vi "Route.vi"(8 "error in (no error)":errorcluster, 9 "Connect":bool, 10 "channel 1":string caption="Route", 11 "reference in":refnum<class "Switch_MotorP5.lvclass">) -> (0 "error out":errorcluster, 3 "reference in":refnum<class "Switch_MotorP5.lvclass">)   [LabVIEW 2022 SP3, in "Switch_MotorP5.lvlib" / "Switch_MotorP5.lvclass"]
uses:
  Switch_MotorP5.lvclass
  5b888fd5-fbae-499d-b477-1edb2fb80a14.vi
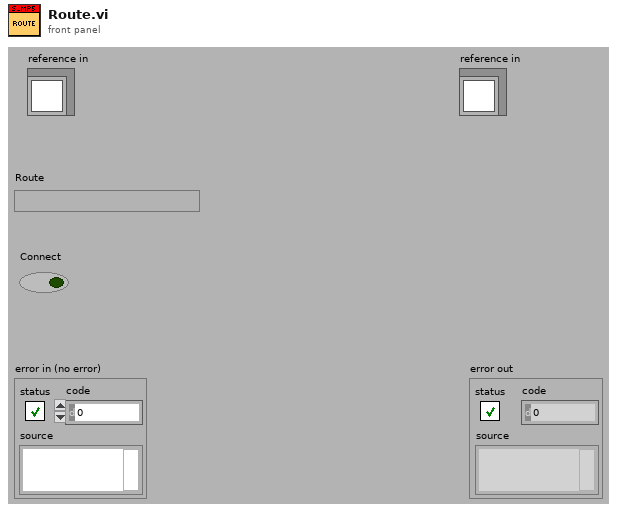
[diagram p1: front panel]
types:
  T1 = typedef "Switch_MotorP5.lvlib/Switch_MotorP5.lvclass/ObjectAttributes.ctl" = cluster{"Config":T2, "VISA":refnum<visa-resource-name>, "RPM":i32, "States":bool[], "UpdateEvent":refnum<user-event>, "Motor":enum32{"M1", "M2", "M3", "M4", "M5", "M6", "M7", "M8"}}
  T2 = typedef "Switch_MotorP5.lvlib/Switch_MotorP5.lvclass/Config.ctl" = cluster{"COM":refnum<visa-resource-name>, "SwitchMap":cluster{"Name":string, "Description":string, "Group":string, "IsGroup":bool, "Motor":enum32{"M1", "M2", "M3", "M4", "M5", "M6", "M7", "M8", "NA"}}[], "Sim":bool}
  T3 = cluster{"Name":string, "Description":string, "Group":string, "IsGroup":bool, "Motor":enum32{"M1", "M2", "M3", "M4", "M5", "M6", "M7", "M8", "NA"}}[]
  T4 = enum32{"M1", "M2", "M3", "M4", "M5", "M6", "M7", "M8", "NA"}
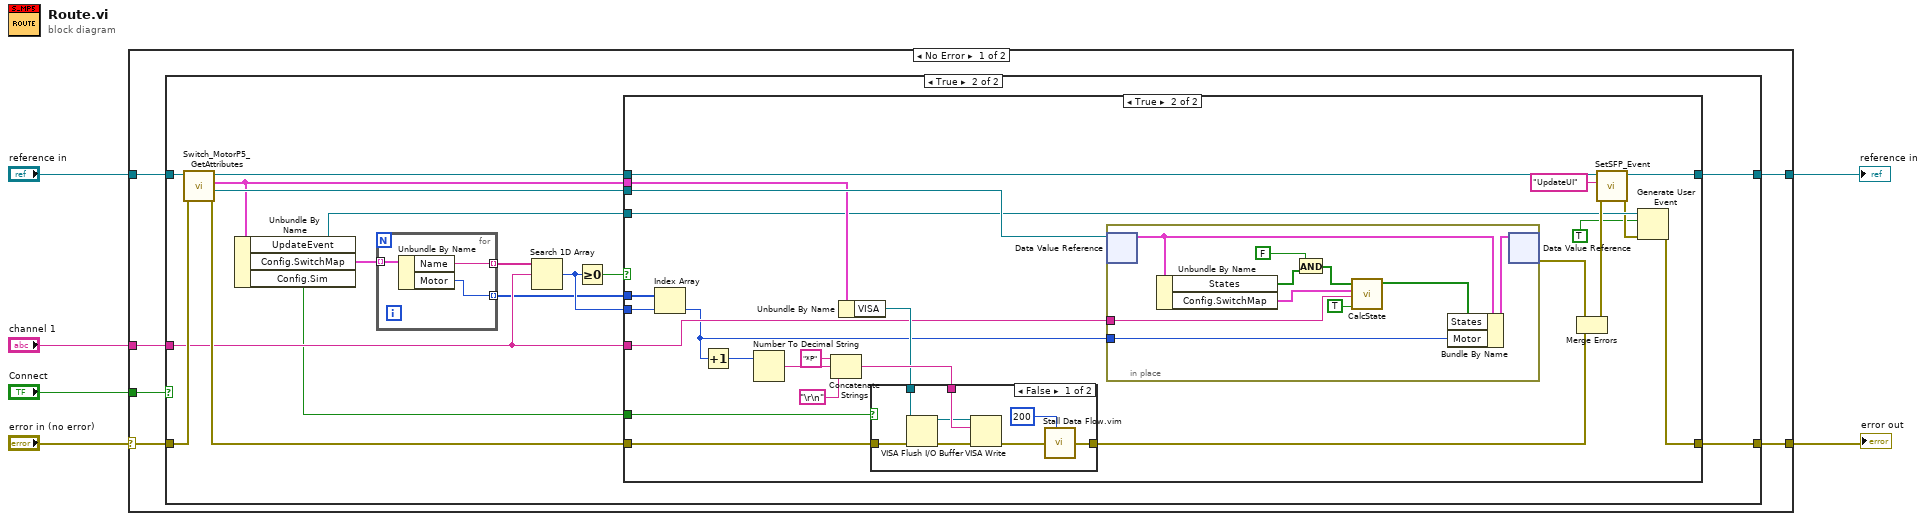
[diagram p0: block diagram]
diagram:
  n1 = case shown="No Error" "error in (no error)" {
    selector: "error in (no error)" -> [w11 w80]
    tunnel: [w8 w80] -> w5
    tunnel: [w9 w79] -> w3
    tunnel: "reference in" -> [w10 w79]
    tunnel: "channel 1" -> [w12 _]
    tunnel: "Connect" -> [w7 _]
    frame No Error {
      n2 = case shown="True" w7 {
        tunnel: w12 -> [_ w20]
        tunnel: w11 -> [w13 w30]
        tunnel: w10 -> [w14 w29]
        tunnel: [w14 w25] -> w9
        tunnel: [w13 w24] -> w8
        frame False {
        }
        frame True {
          n3 = call "Switch_MotorP5_GetAttributes.vi"("error in (no error)"=w30, "reference in"=w29) -> ("error out"=w28:errorcluster, "DataRef"=w27:refnum<data-value>, "Data"=w23:T1, "reference out"=w26:refnum<class "Switch_MotorP5.lvclass">)  [unwired: 6 in]
          n4 = Unbundle By Name(w23) -> ("UpdateEvent"=w15:refnum<user-event>, "Config.SwitchMap"=w22:T3, "Config.Sim"=w16:bool)
          n5 = for {
            tunnel: w22 -> [w78] mode=indexing
            tunnel: [w77] -> w21 mode=indexing
            tunnel: [w76] -> w17 mode=indexing
            n6 = Unbundle By Name(w78) -> ("Name"=w77:string, "Motor"=w76:T4)
          }
          n7 = Search 1D Array(1D array=w21, element=w20) -> (index of element=w18:i32)  [unwired: 1 in]
          n8 = Greater Or Equal To 0?(x=w18) -> (x >= 0?=w19:bool)
          n9 = case shown="True" w19 {
            tunnel: w28 -> [w32 w54]
            tunnel: w27 -> [_ w50]
            tunnel: w26 -> [w31 w49]
            tunnel: [w31 w48] -> w25
            tunnel: [w32 w37] -> w24
            tunnel: w23 -> [_ w43]
            tunnel: w20 -> [_ w35]
            tunnel: w18 -> [_ w42]
            tunnel: w17 -> [_ w41]
            tunnel: w16 -> [_ w40]
            tunnel: w15 -> [_ w39]
            frame False {
            }
            frame True {
              n10 = Index Array(array=w41, index=w42) -> (element=w34:T4)
              n11 = Increment(x=w34) -> (x+1=w33:T4)
              n12 = Number To Decimal String(number=w33) -> (decimal integer string=w56:string)  [unwired: 1 in]
              n13 = Concatenate Strings("*P" ("string"), w56, "\r\n") -> (w55:string)
              n14 = Unbundle By Name(w43) -> ("VISA"=w53:refnum<visa-resource-name>)
              n15 = case shown="False" w40 {
                tunnel: w55 -> [w64 _]
                tunnel: w54 -> [w63 w65]
                tunnel: w53 -> [w61 _]
                tunnel: [w58 w65] -> w44
                frame False {
                  n16 = VISA Flush I/O Buffer(VISA resource name=w61, error in (no error)=w63) -> (VISA resource name out=w60:refnum<visa-resource-name>, error out=w62:errorcluster)  [unwired: 1 in]
                  n17 = VISA Write(VISA resource name=w60, write buffer=w64, error in (no error)=w62) -> (error out=w59:errorcluster)  [unwired: 2 out]
                  n18 = call "Stall Data Flow.vim"("value in"=w59, "milliseconds to wait"=u32 200) -> ("value out"=w58:errorcluster)  [unwired: 1 out]
                }
                frame True {
                }
              }
              n19 = in-place {
                in-place-border: w34 -> [w73]
                in-place-border: w35 -> [w71]
                n20 = in-place-dvr #1(w50) -> (w74:T1)  [unwired: 1 out]
                n21 = Unbundle By Name(w74) -> ("States"=w67:bool[], "Config.SwitchMap"=w72:T3)
                n22 = And(x=FALSE ("State"), y=w67) -> (x .and. y?=w66:bool[])
                n23 = call "CalcState.vi"("State"=TRUE, "Item"=w71, "SwitchMap"=w72, "State_In"=w66) -> ("State_Out"=w69:bool[])  [unwired: 7 in]
                n24 = Bundle By Name(cluster=w74, "States"=w69, "Motor"=w73) -> (w75:T1)
                n25 = in-place-dvr #1(w75) -> (w47:errorcluster)  [unwired: 1 out]
              }
              n26 = Merge Errors(w47, w44) -> (w46:errorcluster)
              n27 = call-dynamic "SetSFP_Event.vi"("error in (no error)"=w46, "msg"="UpdateUI", "reference in"=w49) -> ("error out"=w38:errorcluster, "reference out"=w48:refnum<class "Switch_MotorP5.lvclass">)  [unwired: 7 in]
              n28 = Generate User Event(user event=w39, event data cluster=TRUE, error in=w38) -> (error out=w37:errorcluster)  [unwired: 1 in, 1 out]
            }
          }
        }
      }
    }
    frame Error {
    }
  }
  "error out" <- w5
  "reference in" <- w3
